vi "MainPage.vi"() -> ()   [LabVIEW 2017]
doc: "<B>This VI is using for Capabilities Files parsing and modifying.</B>"
uses:
  API/Parser/Paser.lvlib
  Ctrl/State.ctl
  Ctrl/EnumValue.ctl
  Ctrl/Enum.ctl
  Ctrl/ScaleType.ctl
  Ctrl/Scale.ctl
  Ctrl/Bitfield.ctl
  Ctrl/Register.ctl
  Ctrl/Property.ctl
  Ctrl/PhysicalChannel.ctl
  Ctrl/Caps.ctl
  Ctrl/Data.ctl
panel:
  out "Lable":string
  in  "Open":bool
  in  "Save":bool
  out "Error Output":errorcluster
  in  "confirm":bool
  in  "String":string
  in  "U8":u8 format="%.0x"
  in  "I8":i8
  in  "U32":u32
  in  "I32":i32
  in  "U64":u64
  in  "I64":i64
  in  "Ring":u16(ring) items=["False", "True"]
  in  "DBL":dbl format="%#_16g"
  in  "Add":bool
  in  "Remove":bool
  in  "stop":bool
  in  "Property tree":string[](tree)=["a"]
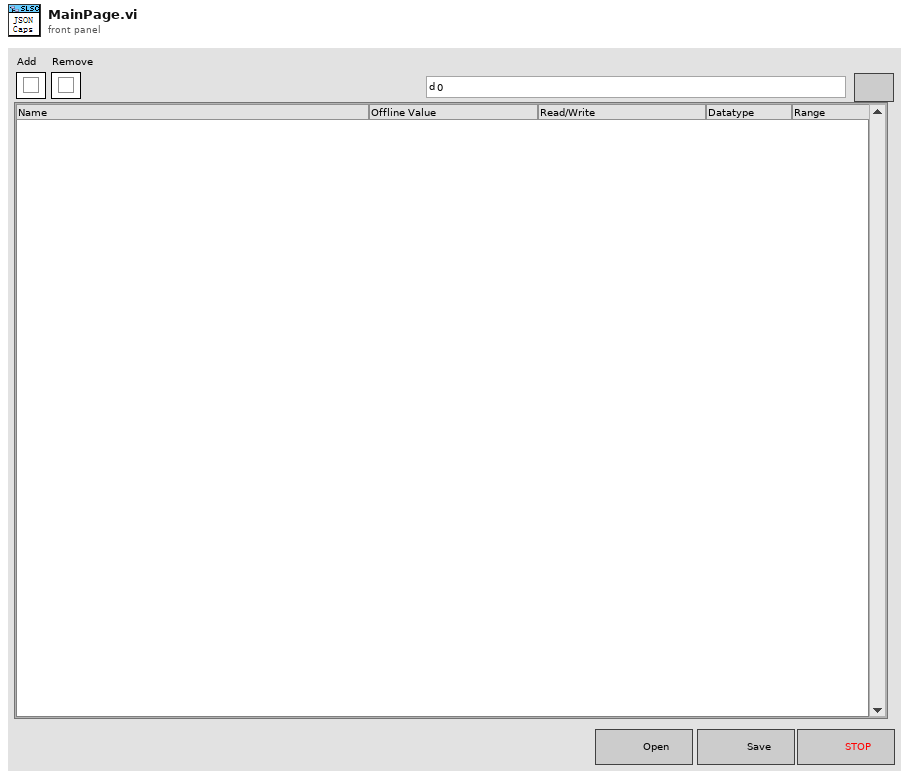
[diagram p1: front panel]
types:
  T1 = typedef "Data.ctl" = cluster{"Ref Cluster":cluster{"String":refnum<vi>, "U8":refnum<vi>, "I8":refnum<vi>, "U32":refnum<vi>, "I32":refnum<vi>, "U64":refnum<vi>, "I64":refnum<vi>, "Ring":refnum<vi>, "DBL":refnum<vi>, "Add":refnum<vi>, "Remove":refnum<vi>, "Property tree":refnum<vi>, "confirm":refnum<vi>}, "JSON Text":string, "Original JSON Text":string, "Caps":T2, "SLSC Output Tree":cluster{"Left Cell String":string, "Child Text":string[], "Child Tag":string, "Item Indent":i32, "Child Only?":bool, "Glyph Index":i32, "offline value":variant}[], "Ref Index and Control Type":cluster{"index":i32, "Datatype":string}, "Selected Type and name":cluster{"Selected Type":enum16{"Property", "Physical Channel", "Other"}, "Selected Property Name":string}, "Update whole Tree?":bool}
  T2 = typedef "Caps.ctl" = cluster{"properties":T3[], "physical channels":T4[], "registers":T5[], "scales":T7[], "enums":T9[], "productName":string}
  T3 = typedef "Property.ctl" = cluster{"name":string, "bitfield":string, "value":variant, "dataType":string, "min":variant, "max":variant, "scale":string, "access":string}
  T4 = typedef "PhysicalChannel.ctl" = cluster{"name":string, "properties":T3[]}
  T5 = typedef "Register.ctl" = cluster{"name":string, "address":i32, "size":i32, "bitfields":T6[], "initialValue":variant, "connectedProperties":string[]}
  T6 = typedef "Bitfield.ctl" = cluster{"name":string, "offset":i32, "size":i32, "signed":bool}
  T7 = typedef "Scale.ctl" = cluster{"name":string, "type":T8, "params":variant}
  T8 = typedef "ScaleType.ctl" = enum16{"NoScale", "Table", "Polynomial", "Linear"}
  T9 = typedef "Enum.ctl" = cluster{"name":string, "values":T10[]}
  T10 = typedef "EnumValue.ctl" = cluster{"name":string, "value":i32}
  T11 = cluster{"String":refnum<vi>, "U8":refnum<vi>, "I8":refnum<vi>, "U32":refnum<vi>, "I32":refnum<vi>, "U64":refnum<vi>, "I64":refnum<vi>, "Ring":refnum<vi>, "DBL":refnum<vi>, "Add":refnum<vi>, "Remove":refnum<vi>, "Property tree":refnum<vi>, "confirm":refnum<vi>}
  T12 = typedef "State.ctl" = enum16{"Initial", "Parse", "Update", "Idle", "Confirm", "Save", "Close", "Add", "Remove"}
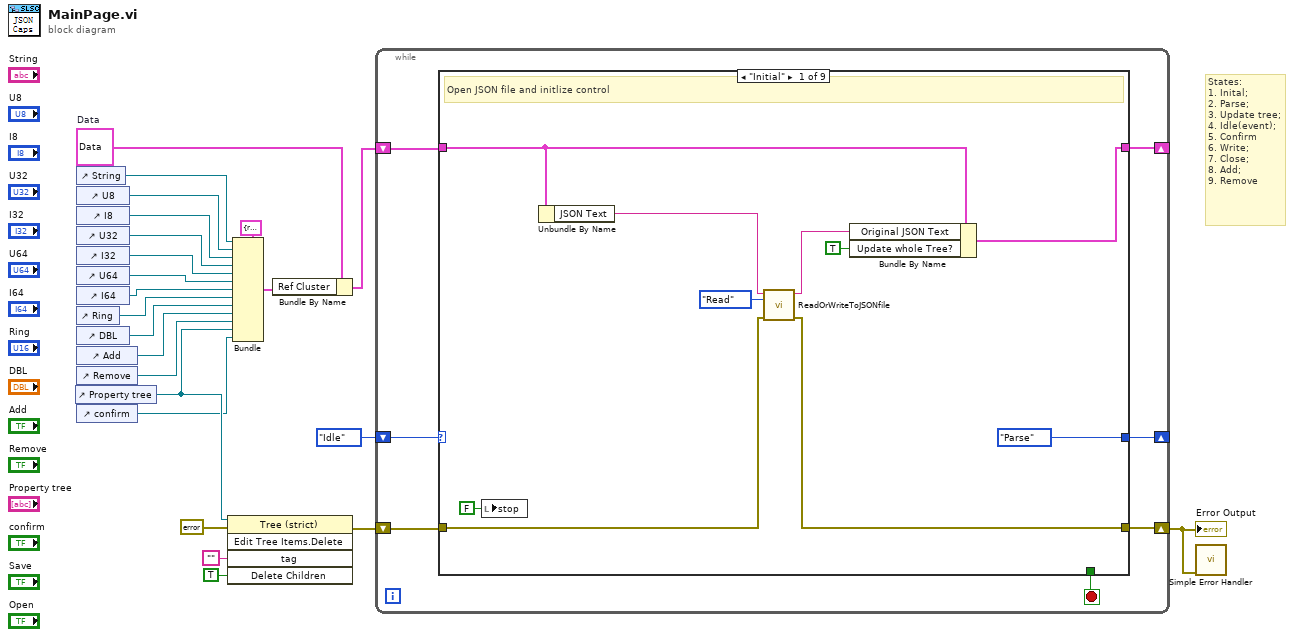
[diagram p0: block diagram]
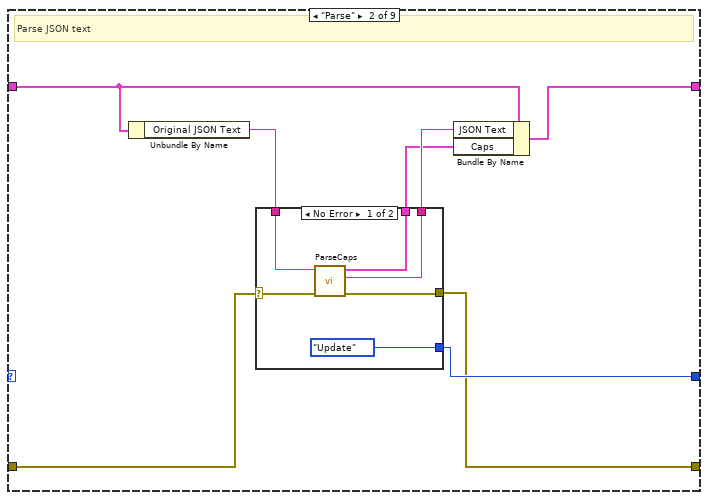
[diagram p2: hidden frame]
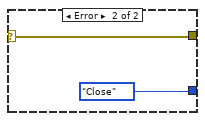
[diagram p3: hidden frame]
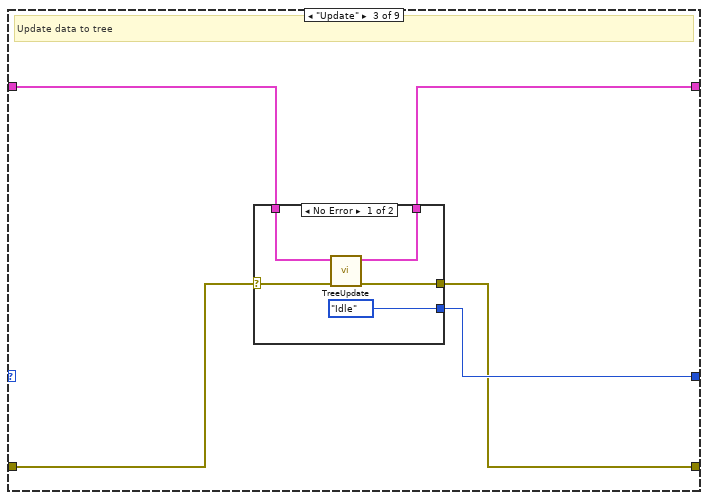
[diagram p4: hidden frame]
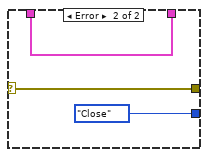
[diagram p5: hidden frame]
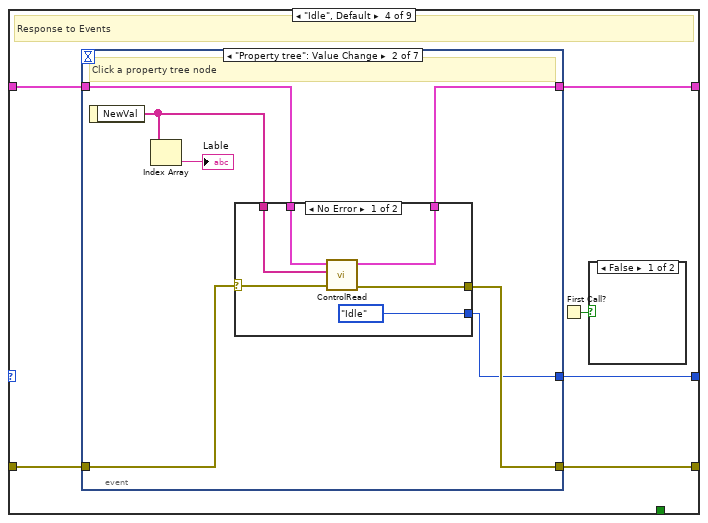
[diagram p6: hidden frame]
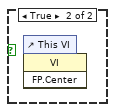
[diagram p7: hidden frame]
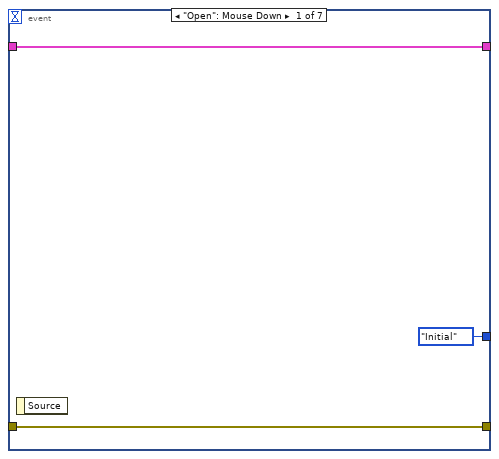
[diagram p8: hidden frame]
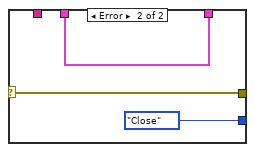
[diagram p9: hidden frame]
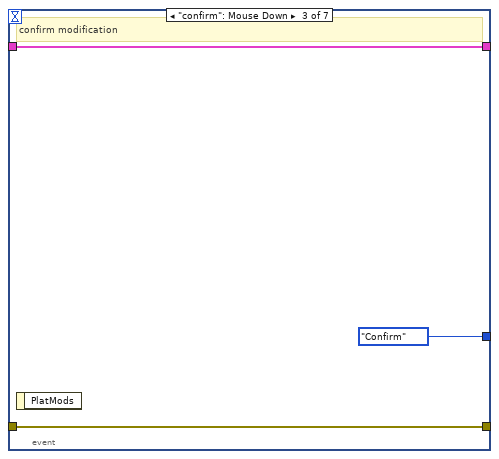
[diagram p10: hidden frame]
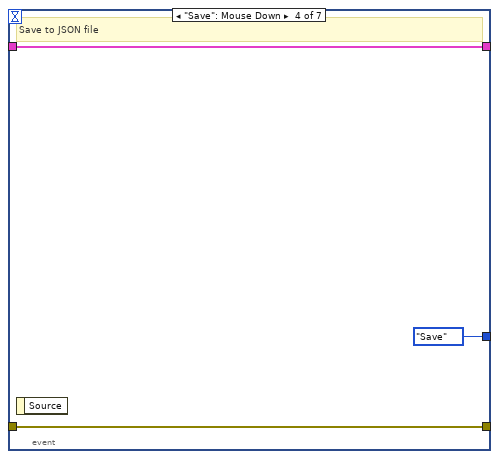
[diagram p11: hidden frame]
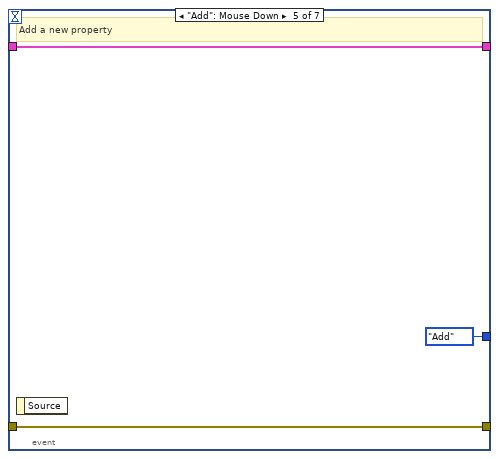
[diagram p12: hidden frame]
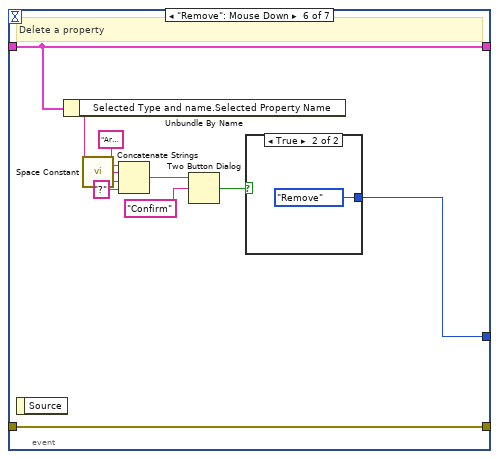
[diagram p13: hidden frame]
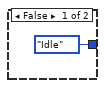
[diagram p14: hidden frame]
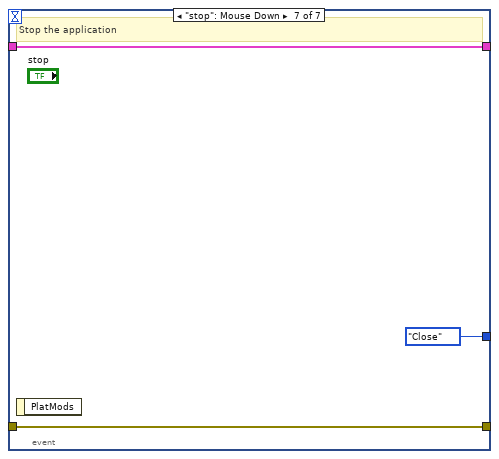
[diagram p15: hidden frame]
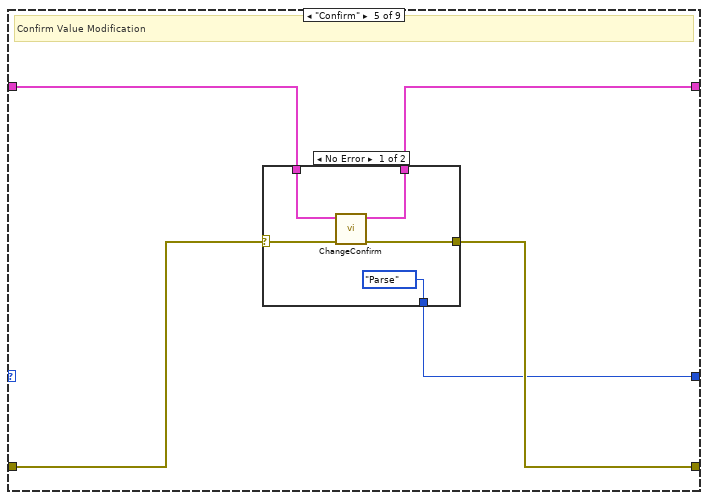
[diagram p16: hidden frame]
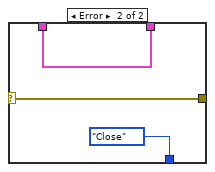
[diagram p17: hidden frame]
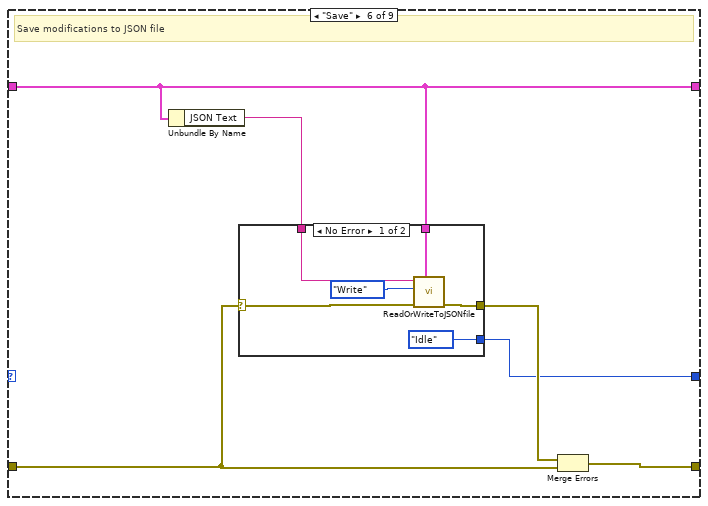
[diagram p18: hidden frame]
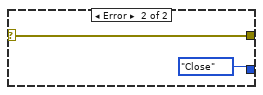
[diagram p19: hidden frame]
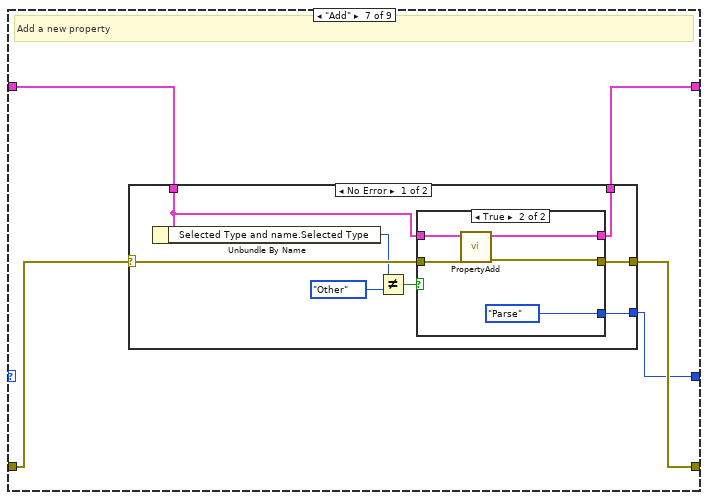
[diagram p20: hidden frame]
diagram:
  w8 = T1 {"Ref Cluster"={"String"=refnum, "U8"=refnum, "I8"=refnum, "U32"=refnum, "I32"=refnum, "U64"=refnum, "I64"=refnum, "Ring"=refnum, "DBL"=refnum, "Add"=refnum, "Remove"=refnum, "Property tree"=refnum, "confirm"=refnum}, "JSON Text"="", "Original JSON Text"="", "Caps"={"properties"=[], "physical channels"=[], "registers"=[], "scales"=[], "enums"=[], "productName"=""}, "SLSC Output Tree"=[], "Ref Index and Control Type"={"index"=0, "Datatype"=""}, "Selected Type and name"={"Selected Type"=enum."Property", "Selected Property Name"=""}, "Update whole Tree?"=FALSE}  # Data
  # "States:\n1. Inital;\n2. Parse;\n3. Update tree;\n4. Idle(event);\n5. Confirm\n6. Write;\n7. Close;\n8. Add;\n9. Remove"
  n1 = control-ref of="Property tree"() -> (w4:refnum<vi>)
  n2 = control-ref of="String"() -> (w22:refnum<vi>)
  n3 = control-ref of="U8"() -> (w21:refnum<vi>)
  n4 = control-ref of="I8"() -> (w20:refnum<vi>)
  n5 = control-ref of="U32"() -> (w19:refnum<vi>)
  n6 = control-ref of="I32"() -> (w18:refnum<vi>)
  n7 = control-ref of="U64"() -> (w17:refnum<vi>)
  n8 = control-ref of="I64"() -> (w16:refnum<vi>)
  n9 = control-ref of="Ring"() -> (w15:refnum<vi>)
  n10 = control-ref of="DBL"() -> (w14:refnum<vi>)
  n11 = control-ref of="Add"() -> (w13:refnum<vi>)
  n12 = control-ref of="Remove"() -> (w12:refnum<vi>)
  n13 = control-ref of="confirm"() -> (w1:refnum<vi>)
  n14 = invoke on="Invoke Node" class="Tree (strict)" method="Edit Tree Items.Delete"(reference=w4, error in=errorcluster {"status"=FALSE, "code"=0, "source"=""} ("error IO"), "tag"="", "Delete Children"=TRUE ("Delete Children?")) -> (error out=w6:errorcluster)  [unwired: 1 in, 4 out]
  n15 = Bundle(cluster=T11 {"String"=refnum, "U8"=refnum, "I8"=refnum, "U32"=refnum, "I32"=refnum, "U64"=refnum, "I64"=refnum, "Ring"=refnum, "DBL"=refnum, "Add"=refnum, "Remove"=refnum, "Property tree"=refnum, "confirm"=refnum}, "String"=w22, "U8"=w21, "I8"=w20, "U32"=w19, "I32"=w18, "U64"=w17, "I64"=w16, "Ring"=w15, "DBL"=w14, "Add"=w13, "Remove"=w12, "Property tree"=w4, "confirm"=w1) -> (w9:T11)
  n16 = Bundle By Name(cluster=w8, "Ref Cluster"=w9) -> (w7:T1)
  n17 = while {
    shift-right: [w29] -> _
    shift-left: State."Idle" -> [w30]
    shift-right: [w24] -> _
    shift-left: w7 -> [w25]
    shift-right: [w26] -> w10
    shift-left: w6 -> [w28]
    stop <- w27 stop-if-true
    n18 = case shown="\"Initial\"" w30 {
      tunnel: [State."Parse" w42 w59 w75 w120 w134 w147 w172 _] -> w29
      tunnel: w25 -> [w32 w45 w61 w74 w124 w133 w151 w174 w187]
      tunnel: [w38 w41 w58 w71 w121 w136 w148 w175 w188] -> w26
      tunnel: w28 -> [w34 w43 w60 w73 w122 w137 w149 w176 w185]
      tunnel: [_ _ _ _ _ _ _ _ TRUE] -> w27
      tunnel: [w39 w46 w57 w72 w123 w133 w150 w173 w187] -> w24
      frame "Initial" {
        # "Open JSON file and initlize control"
        n19 = local write "stop"(FALSE ("Find?")) -> ()
        n20 = Unbundle By Name(w32) -> ("JSON Text"=w31:string)
        n21 = call "ReadOrWriteToJSONfile.vi"("error in (no error)"=w34, "Command"=enum16{"Read", "Write"}."Read" ("Enum"), "JSONtext Input"=w31) -> ("error out"=w38:errorcluster, "JSON text"=w37:string)  [unwired: 7 in]
        n22 = Bundle By Name(cluster=w32, "Original JSON Text"=w37, "Update whole Tree?"=TRUE) -> (w39:T1)
      }
      frame "Parse" {
        # "Parse JSON text"
        n23 = Unbundle By Name(w45) -> ("Original JSON Text"=w44:string)
        n24 = case shown="No Error" w43 {
          selector: w43 -> [w50 w56]
          tunnel: [w54 w56] -> w41
          tunnel: [w53 _] -> w48
          tunnel: [w52 _] -> w47
          tunnel: w44 -> [w51 _]
          tunnel: [State."Update" State."Close"] -> w42
          frame No Error {
            n25 = call "ParseCaps.vi"("error in (no error)"=w50, "caps file text"=w51) -> ("error out"=w54:errorcluster, "json caps"=w53:string, "Caps"=w52:T2)  [unwired: 7 in]
          }
          frame Error {
          }
        }
        n26 = Bundle By Name(cluster=w45, "JSON Text"=w48, "Caps"=w47) -> (w46:T1)
      }
      frame "Update" {
        # "Update data to tree"
        n27 = case shown="No Error" w60 {
          selector: w60 -> [w64 w68]
          tunnel: w61 -> [w66 w69]
          tunnel: [w65 w69] -> w57
          tunnel: [w63 w68] -> w58
          tunnel: [State."Idle" State."Close"] -> w59
          frame No Error {
            n28 = call "TreeUpdate.vi"("error in"=w64, "Data input"=w66) -> ("error out"=w63:errorcluster, "Data output"=w65:T1)  [unwired: 8 in]
          }
          frame Error {
          }
        }
      }
      frame "Idle", Default {
        # "Response to Events"
        n29 = event shown="[1] \"Property tree\": Value Change" {
          selector: _ -> [_ _ _ _ _ _ _]
          dyn-events: _ -> [_ _ _ _ _ _ _]
          timeout: _ -> [_ _ _ _ _ _ _]
          tunnel: [State."Initial" w82 State."Confirm" State."Save" State."Add" w113 State."Close"] -> w75
          tunnel: w74 -> [w78 w86 w98 w101 w104 w112 w118]
          tunnel: [w78 w85 w98 w101 w104 w112 w118] -> w72
          tunnel: [w77 w83 w97 w100 w103 w114 w119] -> w71
          tunnel: w73 -> [w77 w84 w97 w100 w103 w114 w119]
          event "Open": Mouse Down {
            n30 = event-data() -> ()  [unwired: 1 in, 1 out]
          }
          event "Property tree": Value Change {
            # "Click a property tree node"
            n31 = event-data() -> ("NewVal"=w81:string[])  [unwired: 1 in]
            n32 = Index Array(array=w81) -> (element=→"Lable":string)  [unwired: 1 in]
            n33 = case shown="No Error" w84 {
              selector: w84 -> [w89 w94]
              tunnel: w86 -> [w92 w95]
              tunnel: [w91 w95] -> w85
              tunnel: w81 -> [w90 _]
              tunnel: [w88 w94] -> w83
              tunnel: [State."Idle" State."Close"] -> w82
              frame No Error {
                n34 = call "ControlRead.vi"("error in"=w89, "Selected Properties"=w90, "Data input"=w92) -> ("error out"=w88:errorcluster, "Data output"=w91:T1)  [unwired: 7 in]
              }
              frame Error {
              }
            }
          }
          event "confirm": Mouse Down {
            # "confirm modification"
            n35 = event-data() -> ()  [unwired: 1 in, 1 out]
          }
          event "Save": Mouse Down {
            # "Save to JSON file"
            n36 = event-data() -> ()  [unwired: 1 in, 1 out]
          }
          event "Add": Mouse Down {
            # "Add a new property"
            n37 = event-data() -> ()  [unwired: 1 in, 1 out]
          }
          event "Remove": Mouse Down {
            # "Delete a property"
            n38 = event-data() -> ()  [unwired: 1 in, 1 out]
            n39 = Unbundle By Name(w112) -> ("Selected Type and name.Selected Property Name"=w109:string)
            n40 = call <vilib>:"Space Constant.vi"() -> ("String"=w111:string)
            n41 = Concatenate Strings("Are you sure you want to remove" ("string"), w111, w109, "?" ("string")) -> (w107:string)
            n42 = Two Button Dialog(message=w107, 2:"Confirm" ("T button name (\"OK\")")) -> (T button?=w105:bool)  [unwired: 1 in]
            n43 = case shown="True" w105 {
              tunnel: [State."Idle" State."Remove"] -> w113
              frame False {
              }
              frame True {
              }
            }
          }
          event "stop": Mouse Down {
            # "Stop the application"
            n44 = event-data() -> ()  [unwired: 1 in, 1 out]
          }
        }
        n45 = First Call?() -> (First Call?: T/F=w70:bool)
        n46 = case shown="False" w70 {
          frame False {
          }
          frame True {
            n47 = control-ref of="This VI"() -> (w76:refnum<vi>)
            n48 = invoke class="VI" method="FP.Center"(reference=w76) -> ()  [unwired: 2 in, 3 out]
          }
        }
      }
      frame "Confirm" {
        # "Confirm Value Modification"
        n49 = case shown="No Error" w122 {
          selector: w122 -> [w127 w132]
          tunnel: w124 -> [w129 w131]
          tunnel: [w128 w131] -> w123
          tunnel: [w126 w132] -> w121
          tunnel: [State."Parse" State."Close"] -> w120
          frame No Error {
            n50 = call "ChangeConfirm.vi"("error in"=w127, "Data input"=w129) -> ("error out"=w126:errorcluster, "Data ouput"=w128:T1)  [unwired: 8 in]
          }
          frame Error {
          }
        }
      }
      frame "Save" {
        # "Save modifications to JSON file"
        n51 = Unbundle By Name(w133) -> ("JSON Text"=w135:string)
        n52 = case shown="No Error" w137 {
          selector: w137 -> [w140 w146]
          tunnel: [w143 w146] -> w138
          tunnel: w135 -> [w142 _]
          tunnel: [State."Idle" State."Close"] -> w134
          tunnel: w133 -> [w139 _]
          frame No Error {
            n53 = call "ReadOrWriteToJSONfile.vi"("Data"=w139, "error in (no error)"=w140, "Command"=enum16{"Read", "Write"}."Write" ("Enum"), "JSONtext Input"=w142) -> ("error out"=w143:errorcluster)  [unwired: 6 in, 1 out]
          }
          frame Error {
          }
        }
        n54 = Merge Errors(w138, w137) -> (w136:errorcluster)
      }
      frame "Add" {
        # "Add a new property"
        n55 = case shown="No Error" w149 {
          selector: w149 -> [w158 w170]
          tunnel: w151 -> [w152 w169]
          tunnel: [w159 w169] -> w150
          tunnel: [w157 w170] -> w148
          tunnel: [w156 State."Close"] -> w147
          frame No Error {
            n56 = Unbundle By Name(w152) -> ("Selected Type and name.Selected Type"=w154:enum16{"Property", "Physical Channel", "Other"})
            n57 = Not Equal?(x=w154, y=enum16{"Property", "Physical Channel", "Other"}."Other") -> (x != y?=w155:bool)
            n58 = case shown="True" w155 {
              tunnel: [w163 w168] -> w159
              tunnel: w158 -> [w162 w167]
              tunnel: [w162 w166] -> w157
              tunnel: [State."Idle" State."Parse"] -> w156
              tunnel: w152 -> [w163 w164]
              frame False {
                n59 = One Button Dialog(message="Please select a right position to insert.") -> ()  [unwired: 1 in, 1 out]
              }
              frame True {
                n60 = call "PropertyAdd.vi"("error in"=w167, "Data"=w164) -> ("error out"=w166:errorcluster, "Data 2"=w168:T1)  [unwired: 8 in]
              }
            }
          }
          frame Error {
          }
        }
      }
      frame "Remove" {
        # "Remove a property"
        n61 = case shown="No Error" w176 {
          selector: w176 -> [w181 w184]
          tunnel: [w180 w184] -> w175
          tunnel: w174 -> [w179 w183]
          tunnel: [w178 w183] -> w173
          tunnel: [State."Parse" State."Close"] -> w172
          frame No Error {
            n62 = call "PropertyDelete.vi"("Data"=w179, "error in"=w181) -> ("Data 2"=w178:T1, "error out"=w180:errorcluster)  [unwired: 16 in]
          }
          frame Error {
          }
        }
      }
      frame "Close" {
        # "Close all reference"
        n63 = Unbundle By Name(w187) -> ("Ref Cluster.String"=w202:refnum<vi>, "Ref Cluster.U8"=w201:refnum<vi>, "Ref Cluster.I8"=w200:refnum<vi>, "Ref Cluster.U32"=w199:refnum<vi>, "Ref Cluster.I32"=w198:refnum<vi>, "Ref Cluster.U64"=w197:refnum<vi>, "Ref Cluster.I64"=w196:refnum<vi>, "Ref Cluster.Ring"=w195:refnum<vi>, "Ref Cluster.DBL"=w194:refnum<vi>, "Ref Cluster.Add"=w193:refnum<vi>, "Ref Cluster.Remove"=w192:refnum<vi>, "Ref Cluster.Property tree"=w186:refnum<vi>)
        n64 = Build Array(w202, w201, w200, w199, w198, w197, w196, w195, w194, w193, w192, w186) -> (w191:refnum<vi>[])
        n65 = for {
          tunnel: w191 -> [w204] mode=indexing
          tunnel: [w205] -> w189
          tunnel: w185 -> [w203]
          n66 = Close Reference(reference=w204, error in (no error)=w203) -> (error out=w205:errorcluster)
        }
        n67 = Merge Errors(w189, w185) -> (w188:errorcluster)
      }
    }
  }
  "Error Output" <- w10
  n68 = call <vilib>:"Simple Error Handler.vi"("error in (no error)"=w10) -> ()  [unwired: 4 in, 5 out]
